vi "CCE RRMA T030 SubVI01.vi"(10 "CAPA DE COLOR":T1(ring)=enum."RGB2GRAY MATLAB", 11 "Image Pixels (U32)":u32[][](array[numeric])) -> (2 "capa u8":u8[][](array[numeric]), 3 "imagen u32":u32[][](array[numeric]))   [LabVIEW 2020]
doc: "Ceballos Conde Emanuel Rodríguez Ramírez Miguel Ángel 4MV6 Sistemas de visión artificial 2022/1\neste vi permite hacer la conversion obtener una capa de las componentes RGB, HSV,CMY o escala de grisis,"
panel:
  # "Ceballos Conde Emanuel\nRodríguez Ramírez Miguel Ángel\n4MV6\nSistemas de visión artificial\n2022/1"
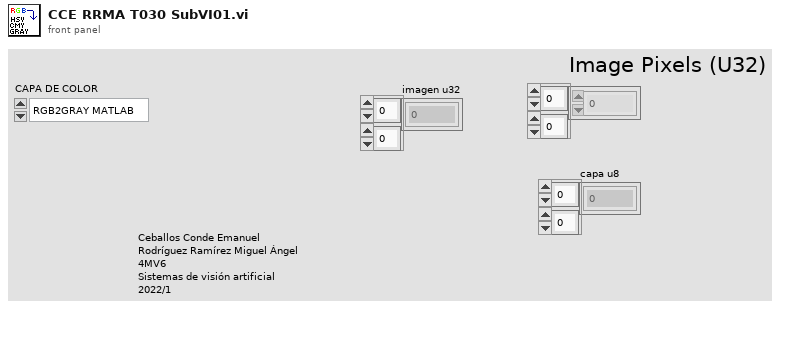
[diagram p1: front panel]
types:
  T1 = enum16{"H", "S", "V", "C", "M", "Y", "R", "G", "B", "RGB2GRAY MATLAB"}
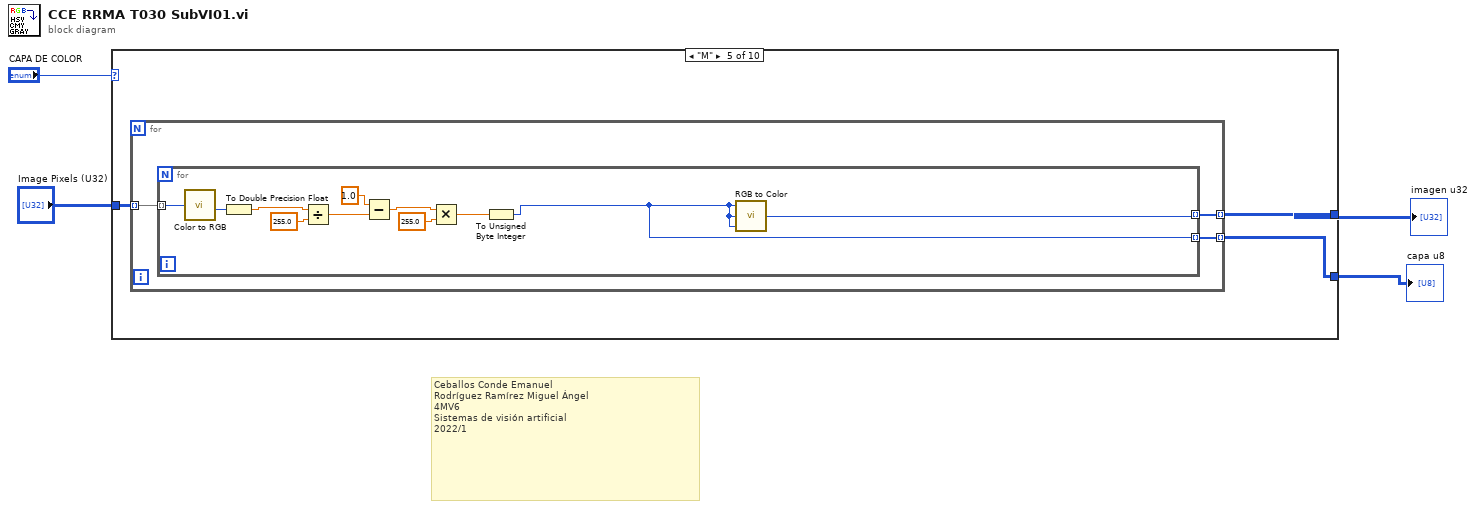
[diagram p0: block diagram]
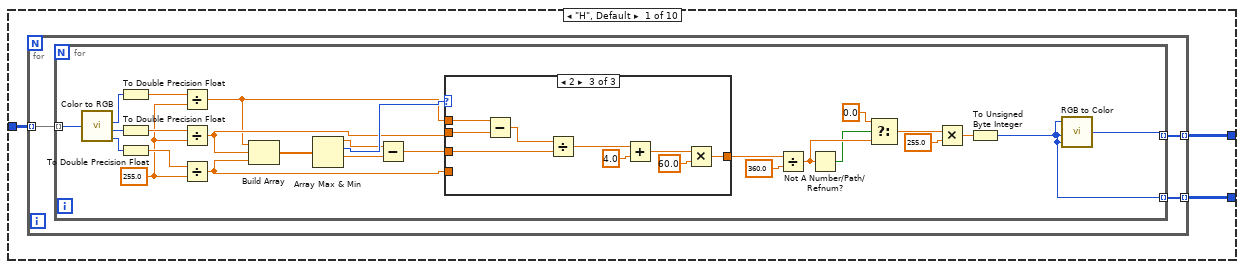
[diagram p2: hidden frame]
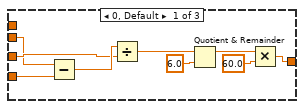
[diagram p3: hidden frame]
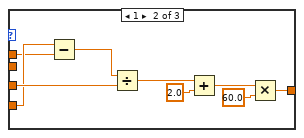
[diagram p4: hidden frame]
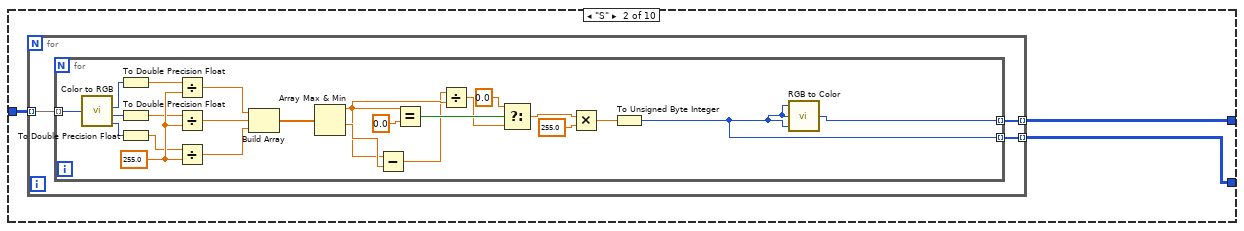
[diagram p5: hidden frame]
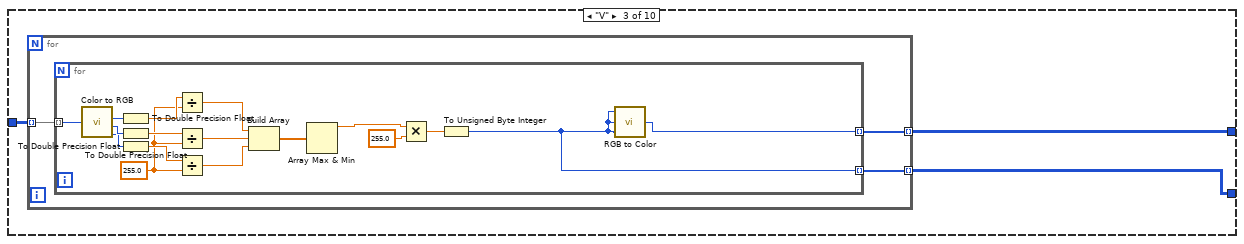
[diagram p6: hidden frame]
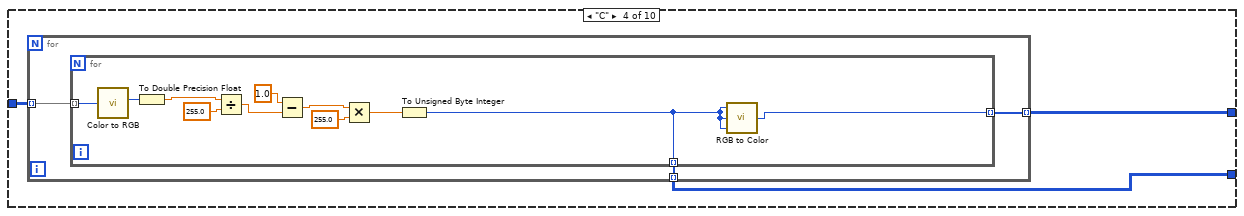
[diagram p7: hidden frame]
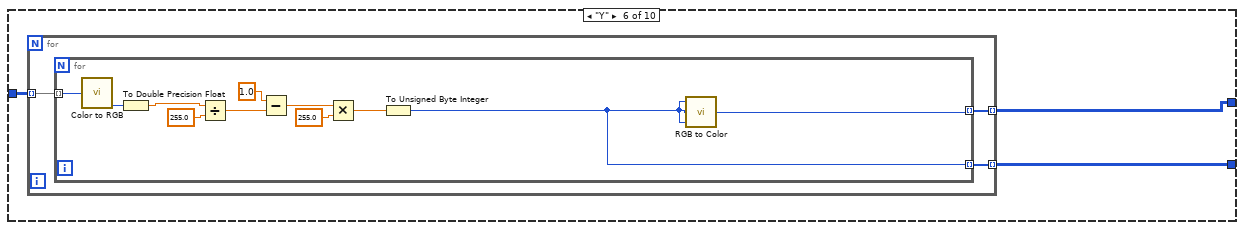
[diagram p8: hidden frame]
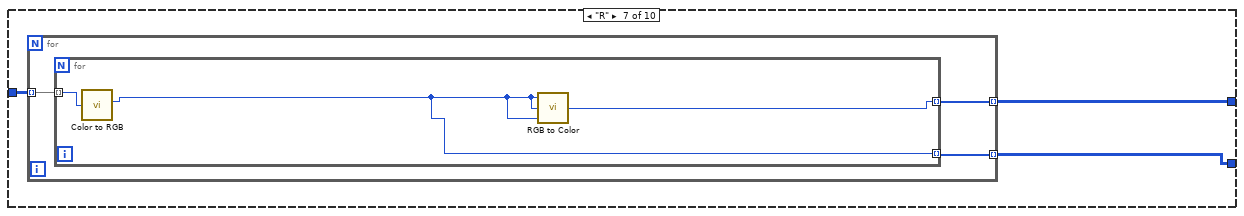
[diagram p9: hidden frame]
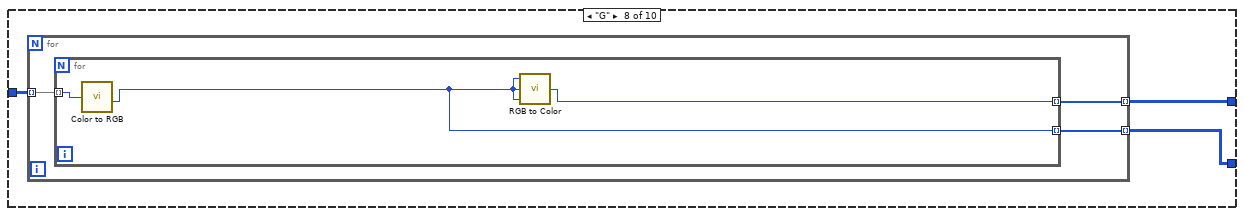
[diagram p10: hidden frame]
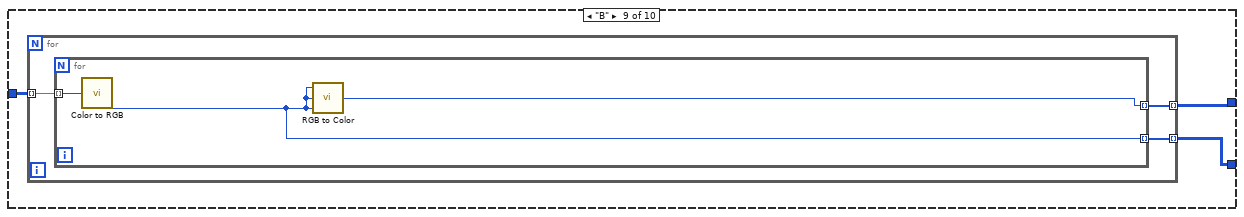
[diagram p11: hidden frame]
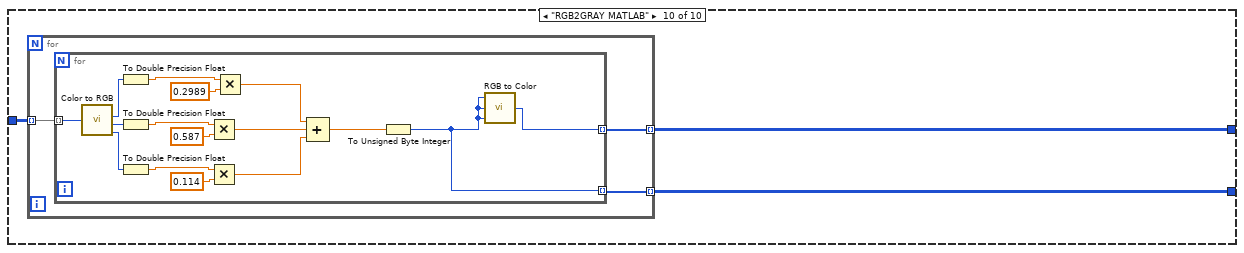
[diagram p12: hidden frame]
diagram:
  # "Ceballos Conde Emanuel\nRodríguez Ramírez Miguel Ángel\n4MV6\nSistemas de visión artificial\n2022/1"
  n1 = case shown="\"M\"" "CAPA DE COLOR" {
    tunnel: [w7 w66 w96 w118 w135 w152 w169 w178 w187 w196] -> w3
    tunnel: "Image Pixels (U32)" -> [w6 w65 w95 w119 w136 w153 w170 w179 w188 w197]
    tunnel: [w5 w64 w94 w117 w134 w151 w168 w177 w186 w195] -> w1
    frame "H", Default {
      n2 = for {
        tunnel: [w10] -> w7 mode=indexing
        tunnel: w6 -> [w9] mode=indexing
        tunnel: [w8] -> w5 mode=indexing
        n3 = for {
          tunnel: [w12] -> w10 mode=indexing
          tunnel: w9 -> [w19] mode=indexing
          tunnel: [w11] -> w8 mode=indexing
          w22 = 255.0 ("y")
          n4 = call <vilib>:"Color to RGB.vi"("Color"=w19) -> ("R"=w18:u8, "G"=w17:u8, "B"=w16:u8)  [unwired: 1 out]
          n5 = To Double Precision Float(number=w18) -> (double precision float=w23:dbl)
          n6 = To Double Precision Float(number=w17) -> (double precision float=w24:dbl)
          n7 = To Double Precision Float(number=w16) -> (double precision float=w25:dbl)
          n8 = Divide(x=w23, y=w22) -> (x/y=w31:dbl)
          n9 = Divide(x=w24, y=w22) -> (x/y=w32:dbl)
          n10 = Divide(x=w25, y=w22) -> (x/y=w33:dbl)
          n11 = Build Array(w31, w32, w33) -> (w26:dbl[])
          n12 = Array Max & Min(array=w26) -> (max value=w28:dbl, max index (indices)=w36:i32, min value=w27:dbl)  [unwired: 1 out]
          n13 = Subtract(x=w28, y=w27) -> (x-y=w29:dbl)
          n14 = case shown="2" w36 {
            tunnel: [w39 w48 w57] -> w30
            tunnel: w32 -> [w38 _ w55]
            tunnel: w33 -> [w37 w47 _]
            tunnel: w29 -> [w44 w53 w62]
            tunnel: w31 -> [_ w46 w56]
            frame 0, Default {
              n15 = Subtract(x=w38, y=w37) -> (x-y=w45:dbl)
              n16 = Divide(x=w45, y=w44) -> (x/y=w43:dbl)
              n17 = Quotient & Remainder(x=w43, y=6.0) -> (x-y*floor(x/y)=w40:dbl)  [unwired: 1 out]
              n18 = Multiply(x=w40, y=60.0) -> (x*y=w39:dbl)
            }
            frame 1 {
              n19 = Subtract(x=w47, y=w46) -> (x-y=w54:dbl)
              n20 = Divide(x=w54, y=w53) -> (x/y=w52:dbl)
              n21 = Add(x=w52, y=2.0) -> (x+y=w49:dbl)
              n22 = Multiply(x=w49, y=60.0) -> (x*y=w48:dbl)
            }
            frame 2 {
              n23 = Subtract(x=w56, y=w55) -> (x-y=w63:dbl)
              n24 = Divide(x=w63, y=w62) -> (x/y=w61:dbl)
              n25 = Add(x=w61, y=4.0) -> (x+y=w58:dbl)
              n26 = Multiply(x=w58, y=60.0) -> (x*y=w57:dbl)
            }
          }
          n27 = Divide(x=w30, y=360.0) -> (x/y=w35:dbl)
          n28 = Not A Number/Path/Refnum?(number/path/refnum=w35) -> (NaN/Path/Refnum?=w34:bool)
          n29 = Select(t=0.0, s=w34, f=w35) -> (s? t:f=w14:dbl)
          n30 = Multiply(x=w14, y=255.0) -> (x*y=w15:dbl)
          n31 = To Unsigned Byte Integer(number=w15) -> (unsigned 8bit integer=w11:u8)
          n32 = call <vilib>:"RGB to Color.vi"("B"=w11, "G"=w11, "R"=w11) -> ("Color"=w12:u32)
        }
      }
    }
    frame "S" {
      n33 = for {
        tunnel: [w69] -> w66 mode=indexing
        tunnel: w65 -> [w68] mode=indexing
        tunnel: [w67] -> w64 mode=indexing
        n34 = for {
          tunnel: [w71] -> w69 mode=indexing
          tunnel: w68 -> [w78] mode=indexing
          tunnel: [w70] -> w67 mode=indexing
          w93 = 255.0 ("y")
          n35 = call <vilib>:"Color to RGB.vi"("Color"=w78) -> ("R"=w77:u8, "G"=w76:u8, "B"=w75:u8)  [unwired: 1 out]
          n36 = To Double Precision Float(number=w77) -> (double precision float=w92:dbl)
          n37 = To Double Precision Float(number=w76) -> (double precision float=w91:dbl)
          n38 = To Double Precision Float(number=w75) -> (double precision float=w90:dbl)
          n39 = Divide(x=w92, y=w93) -> (x/y=w81:dbl)
          n40 = Divide(x=w91, y=w93) -> (x/y=w80:dbl)
          n41 = Divide(x=w90, y=w93) -> (x/y=w79:dbl)
          n42 = Build Array(w81, w80, w79) -> (w89:dbl[])
          n43 = Array Max & Min(array=w89) -> (max value=w83:dbl, min value=w85:dbl)  [unwired: 2 out]
          n44 = Subtract(x=w83, y=w85) -> (x-y=w82:dbl)
          n45 = Equal?(x=w83, y=0.0) -> (x = y?=w87:bool)
          n46 = Divide(x=w82, y=w83) -> (x/y=w84:dbl)
          n47 = Select(t=0.0, s=w87, f=w84) -> (s? t:f=w73:dbl)
          n48 = Multiply(x=w73, y=255.0) -> (x*y=w72:dbl)
          n49 = To Unsigned Byte Integer(number=w72) -> (unsigned 8bit integer=w70:u8)
          n50 = call <vilib>:"RGB to Color.vi"("B"=w70, "G"=w70, "R"=w70) -> ("Color"=w71:u32)
        }
      }
    }
    frame "V" {
      n51 = for {
        tunnel: [w99] -> w96 mode=indexing
        tunnel: w95 -> [w98] mode=indexing
        tunnel: [w97] -> w94 mode=indexing
        n52 = for {
          tunnel: [w101] -> w99 mode=indexing
          tunnel: w98 -> [w108] mode=indexing
          tunnel: [w100] -> w97 mode=indexing
          w110 = 255.0 ("y")
          n53 = call <vilib>:"Color to RGB.vi"("Color"=w108) -> ("R"=w107:u8, "G"=w106:u8, "B"=w105:u8)  [unwired: 1 out]
          n54 = To Double Precision Float(number=w107) -> (double precision float=w111:dbl)
          n55 = To Double Precision Float(number=w106) -> (double precision float=w112:dbl)
          n56 = To Double Precision Float(number=w105) -> (double precision float=w113:dbl)
          n57 = Divide(x=w111, y=w110) -> (x/y=w115:dbl)
          n58 = Divide(x=w112, y=w110) -> (x/y=w109:dbl)
          n59 = Divide(x=w113, y=w110) -> (x/y=w116:dbl)
          n60 = Build Array(w115, w109, w116) -> (w114:dbl[])
          n61 = Array Max & Min(array=w114) -> (max value=w103:dbl)  [unwired: 3 out]
          n62 = Multiply(x=w103, y=255.0) -> (x*y=w102:dbl)
          n63 = To Unsigned Byte Integer(number=w102) -> (unsigned 8bit integer=w100:u8)
          n64 = call <vilib>:"RGB to Color.vi"("B"=w100, "G"=w100, "R"=w100) -> ("Color"=w101:u32)
        }
      }
    }
    frame "C" {
      n65 = for {
        tunnel: w119 -> [w122] mode=indexing
        tunnel: [w121] -> w118 mode=indexing
        tunnel: [w120] -> w117 mode=indexing
        n66 = for {
          tunnel: w122 -> [w133] mode=indexing
          tunnel: [w124] -> w121 mode=indexing
          tunnel: [w123] -> w120 mode=indexing
          n67 = call <vilib>:"Color to RGB.vi"("Color"=w133) -> ("R"=w132:u8)  [unwired: 3 out]
          n68 = To Double Precision Float(number=w132) -> (double precision float=w128:dbl)
          n69 = Divide(x=w128, y=255.0) -> (x/y=w130:dbl)
          n70 = Subtract(x=1.0, y=w130) -> (x-y=w127:dbl)
          n71 = Multiply(x=w127, y=255.0) -> (x*y=w125:dbl)
          n72 = To Unsigned Byte Integer(number=w125) -> (unsigned 8bit integer=w123:u8)
          n73 = call <vilib>:"RGB to Color.vi"("B"=w123, "G"=w123, "R"=w123) -> ("Color"=w124:u32)
        }
      }
    }
    frame "M" {
      n74 = for {
        tunnel: w136 -> [w139] mode=indexing
        tunnel: [w138] -> w135 mode=indexing
        tunnel: [w137] -> w134 mode=indexing
        n75 = for {
          tunnel: w139 -> [w150] mode=indexing
          tunnel: [w141] -> w138 mode=indexing
          tunnel: [w140] -> w137 mode=indexing
          n76 = call <vilib>:"Color to RGB.vi"("Color"=w150) -> ("G"=w142:u8)  [unwired: 3 out]
          n77 = To Double Precision Float(number=w142) -> (double precision float=w146:dbl)
          n78 = Divide(x=w146, y=255.0) -> (x/y=w148:dbl)
          n79 = Subtract(x=1.0, y=w148) -> (x-y=w145:dbl)
          n80 = Multiply(x=w145, y=255.0) -> (x*y=w143:dbl)
          n81 = To Unsigned Byte Integer(number=w143) -> (unsigned 8bit integer=w140:u8)
          n82 = call <vilib>:"RGB to Color.vi"("B"=w140, "G"=w140, "R"=w140) -> ("Color"=w141:u32)
        }
      }
    }
    frame "Y" {
      n83 = for {
        tunnel: w153 -> [w156] mode=indexing
        tunnel: [w155] -> w152 mode=indexing
        tunnel: [w154] -> w151 mode=indexing
        n84 = for {
          tunnel: w156 -> [w167] mode=indexing
          tunnel: [w158] -> w155 mode=indexing
          tunnel: [w157] -> w154 mode=indexing
          n85 = call <vilib>:"Color to RGB.vi"("Color"=w167) -> ("B"=w159:u8)  [unwired: 3 out]
          n86 = To Double Precision Float(number=w159) -> (double precision float=w163:dbl)
          n87 = Divide(x=w163, y=255.0) -> (x/y=w165:dbl)
          n88 = Subtract(x=1.0, y=w165) -> (x-y=w162:dbl)
          n89 = Multiply(x=w162, y=255.0) -> (x*y=w160:dbl)
          n90 = To Unsigned Byte Integer(number=w160) -> (unsigned 8bit integer=w157:u8)
          n91 = call <vilib>:"RGB to Color.vi"("B"=w157, "G"=w157, "R"=w157) -> ("Color"=w158:u32)
        }
      }
    }
    frame "R" {
      n92 = for {
        tunnel: w170 -> [w173] mode=indexing
        tunnel: [w172] -> w169 mode=indexing
        tunnel: [w171] -> w168 mode=indexing
        n93 = for {
          tunnel: w173 -> [w176] mode=indexing
          tunnel: [w175] -> w172 mode=indexing
          tunnel: [w174] -> w171 mode=indexing
          n94 = call <vilib>:"Color to RGB.vi"("Color"=w176) -> ("R"=w174:u8)  [unwired: 3 out]
          n95 = call <vilib>:"RGB to Color.vi"("B"=w174, "G"=w174, "R"=w174) -> ("Color"=w175:u32)
        }
      }
    }
    frame "G" {
      n96 = for {
        tunnel: w179 -> [w182] mode=indexing
        tunnel: [w181] -> w178 mode=indexing
        tunnel: [w180] -> w177 mode=indexing
        n97 = for {
          tunnel: w182 -> [w185] mode=indexing
          tunnel: [w184] -> w181 mode=indexing
          tunnel: [w183] -> w180 mode=indexing
          n98 = call <vilib>:"Color to RGB.vi"("Color"=w185) -> ("G"=w183:u8)  [unwired: 3 out]
          n99 = call <vilib>:"RGB to Color.vi"("B"=w183, "G"=w183, "R"=w183) -> ("Color"=w184:u32)
        }
      }
    }
    frame "B" {
      n100 = for {
        tunnel: w188 -> [w191] mode=indexing
        tunnel: [w190] -> w187 mode=indexing
        tunnel: [w189] -> w186 mode=indexing
        n101 = for {
          tunnel: w191 -> [w194] mode=indexing
          tunnel: [w193] -> w190 mode=indexing
          tunnel: [w192] -> w189 mode=indexing
          n102 = call <vilib>:"Color to RGB.vi"("Color"=w194) -> ("B"=w192:u8)  [unwired: 3 out]
          n103 = call <vilib>:"RGB to Color.vi"("B"=w192, "G"=w192, "R"=w192) -> ("Color"=w193:u32)
        }
      }
    }
    frame "RGB2GRAY MATLAB" {
      n104 = for {
        tunnel: w197 -> [w200] mode=indexing
        tunnel: [w199] -> w196 mode=indexing
        tunnel: [w198] -> w195 mode=indexing
        n105 = for {
          tunnel: w200 -> [w216] mode=indexing
          tunnel: [w202] -> w199 mode=indexing
          tunnel: [w201] -> w198 mode=indexing
          n106 = call <vilib>:"Color to RGB.vi"("Color"=w216) -> ("R"=w215:u8, "G"=w214:u8, "B"=w213:u8)  [unwired: 1 out]
          n107 = To Double Precision Float(number=w215) -> (double precision float=w205:dbl)
          n108 = To Double Precision Float(number=w214) -> (double precision float=w204:dbl)
          n109 = To Double Precision Float(number=w213) -> (double precision float=w203:dbl)
          n110 = Multiply(x=w204, y=0.587) -> (x*y=w208:dbl)
          n111 = Multiply(x=w203, y=0.114) -> (x*y=w207:dbl)
          n112 = Multiply(x=w205, y=0.2989) -> (x*y=w209:dbl)
          n113 = Compound Arithmetic op=ADD(w209, w208, w207) -> (w206:dbl)
          n114 = To Unsigned Byte Integer(number=w206) -> (unsigned 8bit integer=w201:u8)
          n115 = call <vilib>:"RGB to Color.vi"("B"=w201, "G"=w201, "R"=w201) -> ("Color"=w202:u32)
        }
      }
    }
  }
  "imagen u32" <- w3
  "capa u8" <- w1
